vi "convertDeviceData.vi"   [LabVIEW 2011]
uses:
  GlobalVariables.vi
types:
  T1 = typedef "Device Cluster.ctl" = cluster{"Dnet":string, "Node":i32, "Type":string, "ID Number":u8, "SCCM":dbl, "FullScale":dbl, "Input Bytes":i32, "Output Bytes":i32, "Input Start Location":i32, "Output Start Location":i32, "Enabled":bool, "Bytes":u8[]}
  T2 = cluster{"[0]":u8, "[1]":u8, "[2]":u8, "[3]":u8, "[4]":u8, "[5]":u8, "[6]":u8, "[7]":u8}
  T3 = typedef "MFC Cluster.ctl" = cluster{"ID Number":u8, "Status":bool[], "Flow (SCCM)":dbl, "SetPoint (SCCM)":dbl, "Actuator Override":i8, "Actuator Drive Valve":i16, "Setpoint Output":dbl}
  T4 = typedef "PC Cluster.ctl" = cluster{"ID Number":u8, "Status":bool[], "Flow (SCCM)":dbl, "SetPoint (SCCM)":dbl, "Actuator Override":i8, "Actuator Drive Valve":i16, "Setpoint Output":dbl}
  T5 = typedef "RTPC Cluster.ctl" = cluster{"ID Number":u8, "Status":bool[], "Flow (SCCM)":dbl, "Pressure (SCCM)":dbl, "Valve":i16, "Active Instance":i8, "Output":dbl}
  T6 = typedef "GP275 Cluster.ctl" = cluster{"Pressure (Torr)":sgl}
  T7 = typedef "GP354 Cluster.ctl" = cluster{"Degas":bool, "Enable Filament 1":bool, "Enable Filament 2":bool, "Medium Emission":bool, "Ion Gauge":bool, "High Emission":bool, "Pressure":dbl}
  T8 = typedef "BAR Cluster.ctl" = cluster{"Pressure":dbl}
  T9 = typedef "EZ-ZONE Input Cluster.ctl" = cluster{"Device Status":u32, "Analog Input Value 1":sgl, "Analog Input Value 2":sgl, "Heat Power":sgl, "Cool Power":sgl, "Profile Start":u32, "Current Profile":u32, "Current Step":u32, "Active Set Point":sgl, "Step Time Remaining":u32, "Analog Input Error 1":u32, "Analog Input Error 2":u32, "Alarm State 1":u32, "Alarm State 2":u32, "Alarm State 3":u32, "Alarm State 4":u32, "Digital Input Status 5":u32, "Digital Input Status 6":u32, "Control Mode Active":u32, "Limit State":u32, "Profile Action Request":u32}
  T10 = typedef "EZ-ZONE Output Cluster.ctl" = cluster{"Loop Control Mode":u32, "Closed Loop Set Point":sgl, "Open Loop Set Point":sgl, "Alarm 1 - High Set Point":sgl, "Alarm 1 - Low Set Point":sgl, "Alarm 2 - High Set Point":sgl, "Alarm 2 - Low Set Point":sgl, "Alarm 3 - High Set Point":sgl, "Alarm 3 - Low Set Point":sgl, "Alarm 4 - High Set Point":sgl, "Alarm 4 - Low Set Point":sgl, "Profile Action Request":u32, "Profile Start":u32, "Heat Proportional Band":sgl, "Cool Proportional Band":sgl, "Time Integral":sgl, "Time Derivative":sgl, "Heat Hysteresis":sgl, "Cool Hysteresis":sgl, "Dead Band":sgl}
  T11 = typedef "TurboMotor Response Cluster.ctl" = cluster{"Enable":bool, "Index Level":bool, "Current Direction":bool, "General Fault":bool, "Profile in Progress":bool, "Load Complete":bool, "FE Fault":bool, "Rev Limit":bool, "Fwd Limit":bool, "Axis Number":u8, "Message Type":u16, "Data":u8[]}
  T12 = typedef "TurboMotor Command Cluster.ctl" = cluster{"Enable":bool, "Hard Stop":bool, "Smooth Stop":bool, "Direction":bool, "Incremental":bool, "Load Data/Start Profile":bool, "Axis Number":u8, "Message Type":u16, "Data":u8[]}
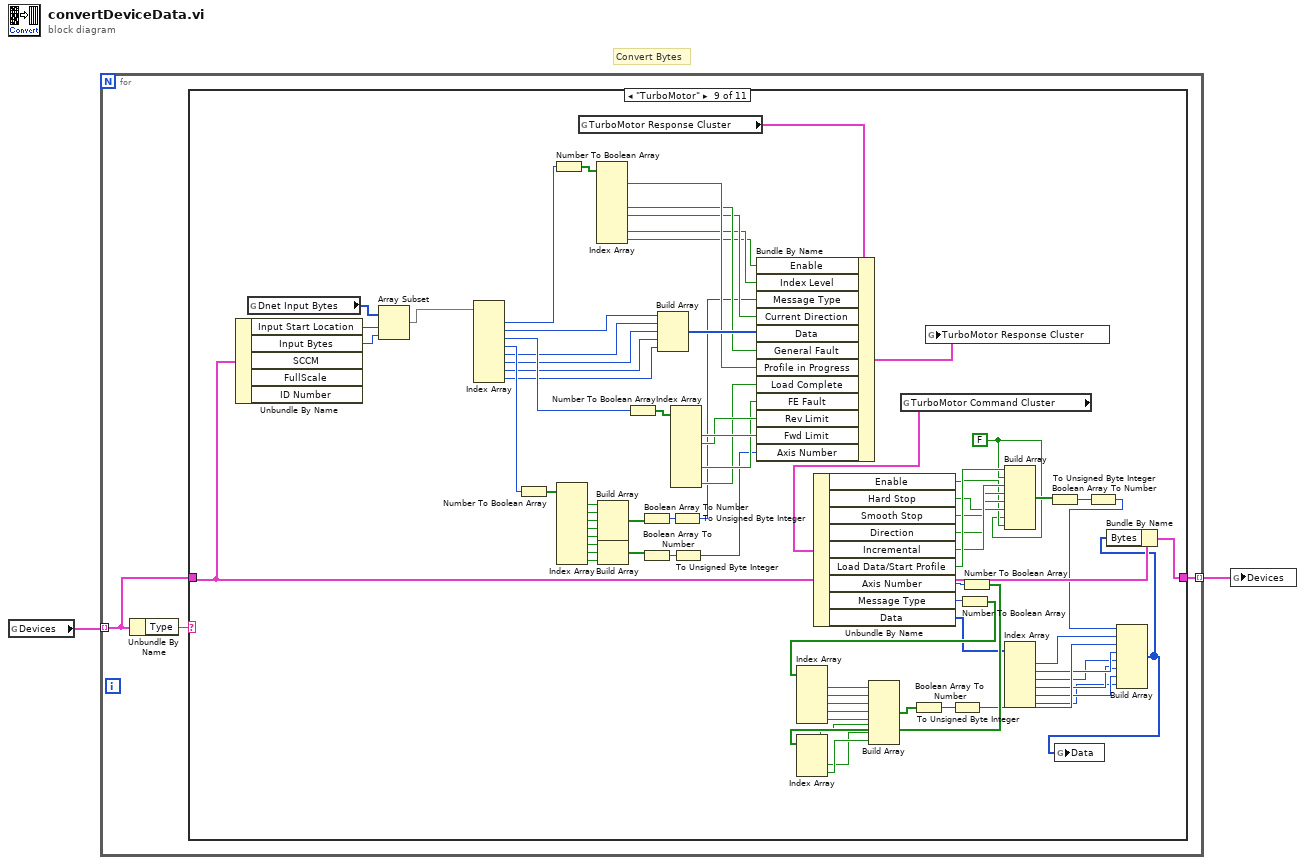
[diagram p0: block diagram]
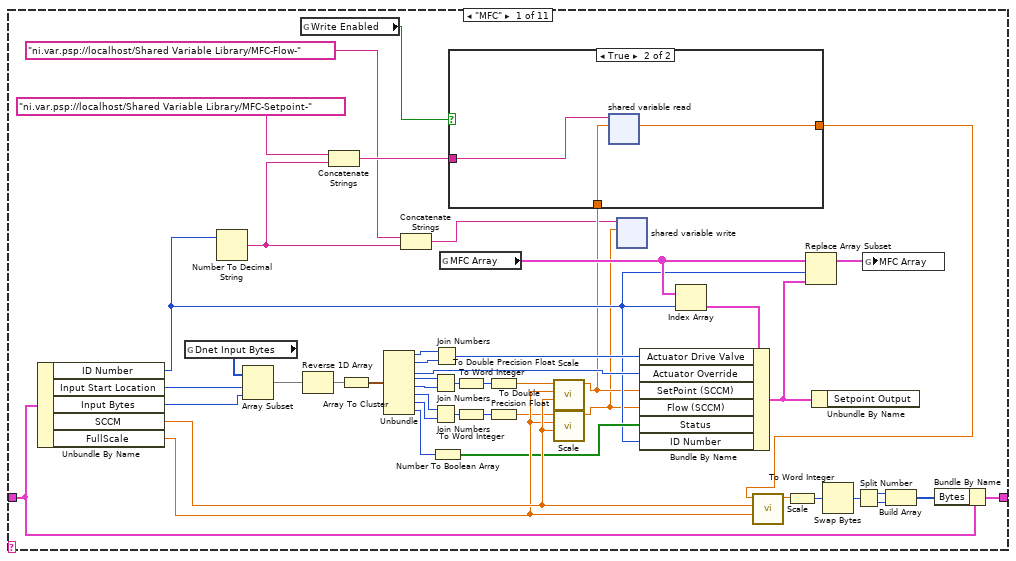
[diagram p2: hidden frame]
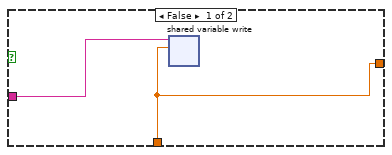
[diagram p3: hidden frame]
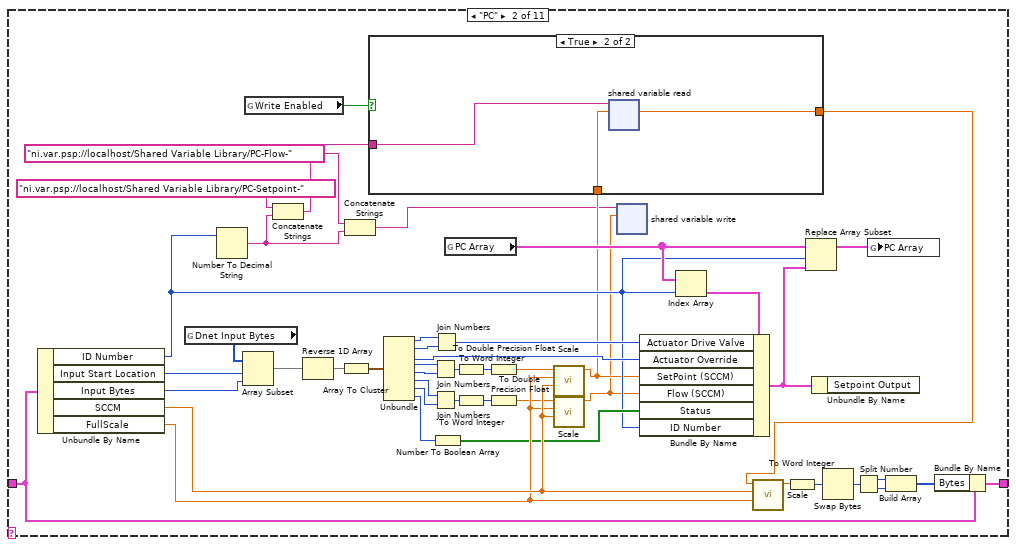
[diagram p4: hidden frame]
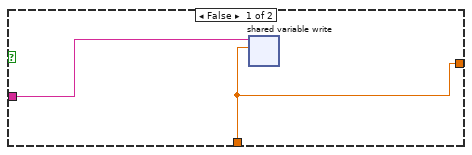
[diagram p5: hidden frame]
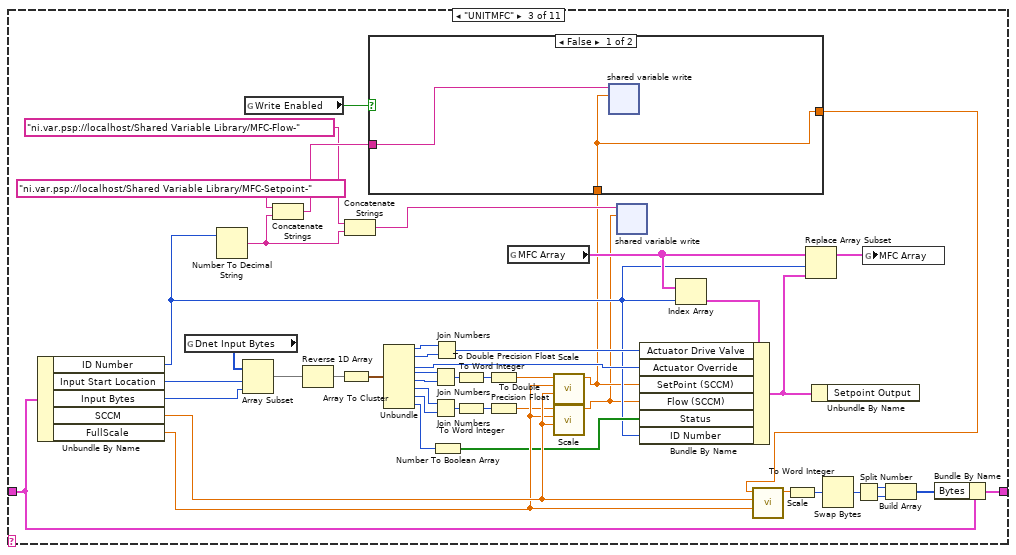
[diagram p6: hidden frame]
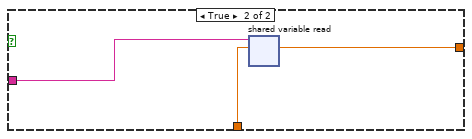
[diagram p7: hidden frame]
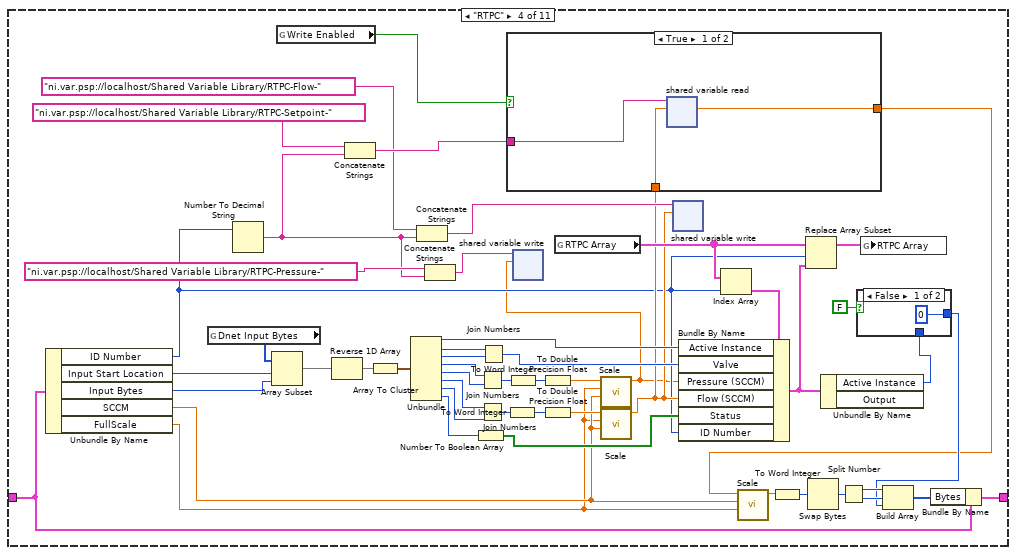
[diagram p8: hidden frame]
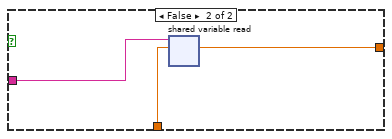
[diagram p9: hidden frame]
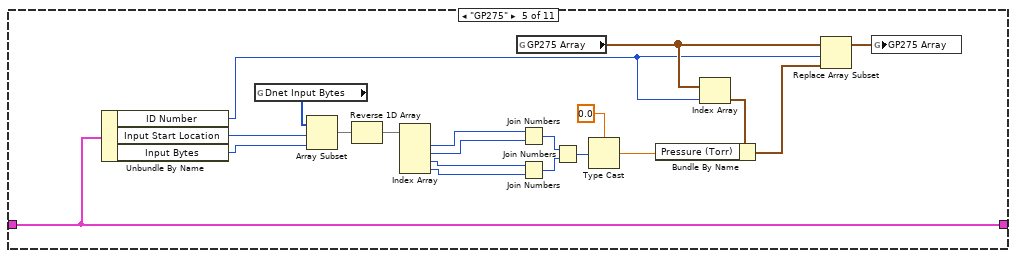
[diagram p11: hidden frame]
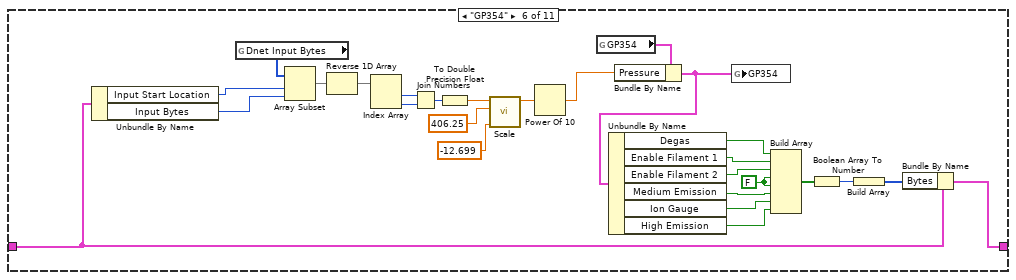
[diagram p12: hidden frame]
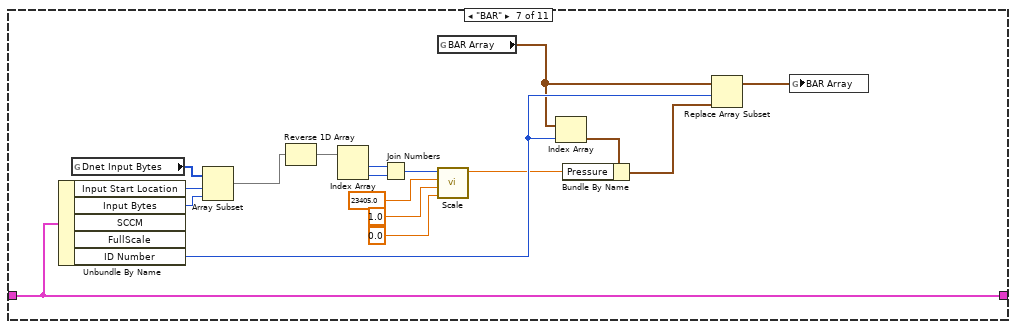
[diagram p13: hidden frame]
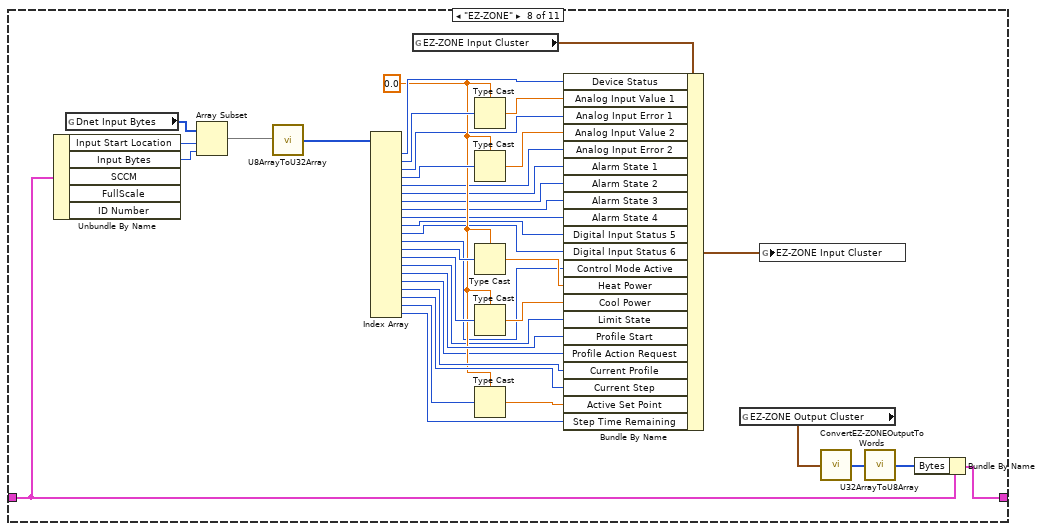
[diagram p14: hidden frame]
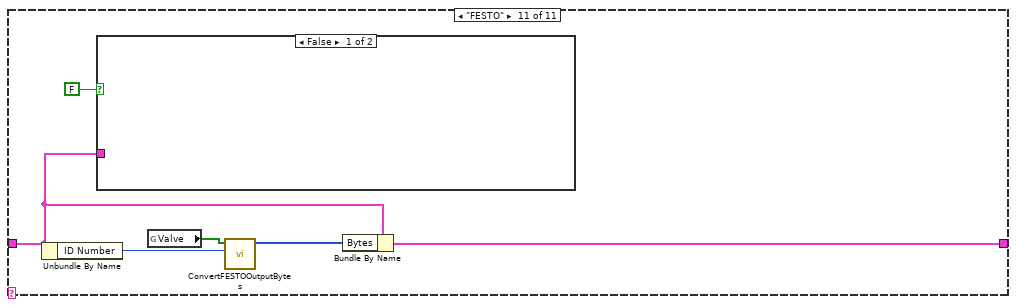
[diagram p16: hidden frame]
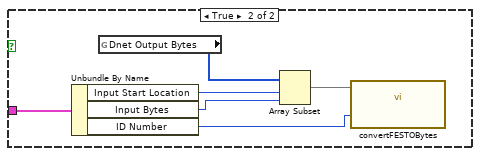
[diagram p17: hidden frame]
diagram:
  # "Convert Bytes"
  n1 = global read "GlobalVariables.vi" "Devices"() -> (w2:T1[])
  n2 = for {
    tunnel: w2 -> [w5] mode=indexing
    tunnel: [w3] -> w1 mode=indexing
    n3 = Unbundle By Name(w5) -> ("Type"=w4:string)
    n4 = case shown="\"TurboMotor\"" w4 {
      tunnel: w5 -> [w16 w67 w118 w174 w218 w262 w276 w283 w365 w399 w402]
      tunnel: [w17 w68 w119 w175 w218 w263 w276 w284 w364 w399 w401] -> w3
      frame "MFC" {
        n5 = Unbundle By Name(w16) -> ("ID Number"=w14:u8, "Input Start Location"=w51:i32, "Input Bytes"=w50:i32, "SCCM"=w49:dbl, "FullScale"=w48:dbl)
        n6 = global read "GlobalVariables.vi" "Dnet Input Bytes"() -> (w31:u8[])
        n7 = Number To Decimal String(number=w14) -> (decimal integer string=w8:string)  [unwired: 1 in]
        n8 = Array Subset(array=w31, index=w51, length=w50) -> (w32:u8[])
        n9 = global read "GlobalVariables.vi" "Write Enabled"() -> (w15:bool)
        n10 = Reverse 1D Array(array=w32) -> (reversed array=w19:u8[])
        n11 = Concatenate Strings("ni.var.psp://localhost/Shared Variable Library/MFC-Setpoint-", w8) -> (w12:string)
        n12 = Array To Cluster(array=w19) -> (cluster=w18:T2)
        n13 = Unbundle(w18) -> ("[0]"=w26:u8, "[1]"=w25:u8, "[2]"=w34:u8, "[3]"=w24:u8, "[4]"=w23:u8, "[5]"=w22:u8, "[6]"=w21:u8, "[7]"=w20:u8)
        n14 = Concatenate Strings("ni.var.psp://localhost/Shared Variable Library/MFC-Flow-", w8) -> (w7:string)
        n15 = Join Numbers(hi=w24, lo=w23) -> ((hi.lo)=w30:u16)
        n16 = Join Numbers(hi=w22, lo=w21) -> ((hi.lo)=w29:u16)
        n17 = Join Numbers(hi=w26, lo=w25) -> ((hi.lo)=w35:u16)
        n18 = Number To Boolean Array(number=w20) -> (Boolean array=w33:bool[])
        n19 = global read "GlobalVariables.vi" "MFC Array"() -> (w38:T3[])
        n20 = To Word Integer(number=w30) -> (16bit integer=w27:i16)
        n21 = To Word Integer(number=w29) -> (16bit integer=w28:i16)
        n22 = To Double Precision Float(number=w27) -> (double precision float=w40:dbl)
        n23 = To Double Precision Float(number=w28) -> (double precision float=w41:dbl)
        n24 = call "Scale.vi"("Factor"=w49, "FullScale"=w48, "Input"=w40) -> ("Output"=w11:dbl)  [unwired: 8 in]
        n25 = case shown="True" w15 {
          tunnel: w12 -> [w53 w56]
          tunnel: w11 -> [w52 w54]
          tunnel: [w52 w55] -> w10
          frame False {
            n26 = shared-variable-write(w53, w52) -> ()  [unwired: 1 in, 2 out]
          }
          frame True {
            n27 = shared-variable-read(w56, w54) -> (w55:dbl)  [unwired: 1 in, 3 out]
          }
        }
        n28 = call "Scale.vi"("Factor"=w49, "FullScale"=w48, "Input"=w41) -> ("Output"=w6:dbl)  [unwired: 8 in]
        n29 = shared-variable-write(w7, w6) -> ()  [unwired: 1 in, 2 out]
        n30 = Index Array(array=w38, index=w14) -> (element=w36:T3)
        n31 = Bundle By Name(cluster=w36, "Actuator Drive Valve"=w35, "Actuator Override"=w34, "SetPoint (SCCM)"=w11, "Flow (SCCM)"=w6, "Status"=w33, "ID Number"=w14) -> (w37:T3)
        n32 = call "Scale.vi"("Factor"=w48, "FullScale"=w49, "Input"=w10) -> ("Output"=w42:dbl)  [unwired: 8 in]
        n33 = To Word Integer(number=w42) -> (16bit integer=w43:i16)
        n34 = Replace Array Subset(array=w38, new element=w37, index=w14) -> (w39:T3[])
        n35 = Unbundle By Name(w37) -> ()  [unwired: 1 out]
        n36 = Swap Bytes(anything=w43) -> (byte swapped=w44:i16)
        n37 = Split Number(x=w44) -> (hi(x)=w46:u8, lo(x)=w45:u8)
        n38 = global write "GlobalVariables.vi" "MFC Array"(w39) -> ()
        n39 = Build Array(w46, w45) -> (w47:u8[])
        n40 = Bundle By Name(cluster=w16, "Bytes"=w47) -> (w17:T1)
      }
      frame "PC" {
        n41 = Unbundle By Name(w67) -> ("ID Number"=w65:u8, "Input Start Location"=w102:i32, "Input Bytes"=w101:i32, "SCCM"=w100:dbl, "FullScale"=w99:dbl)
        n42 = global read "GlobalVariables.vi" "Dnet Input Bytes"() -> (w82:u8[])
        n43 = Number To Decimal String(number=w65) -> (decimal integer string=w59:string)  [unwired: 1 in]
        n44 = Array Subset(array=w82, index=w102, length=w101) -> (w83:u8[])
        n45 = global read "GlobalVariables.vi" "Write Enabled"() -> (w66:bool)
        n46 = Concatenate Strings("ni.var.psp://localhost/Shared Variable Library/PC-Setpoint-", w59) -> (w63:string)
        n47 = Reverse 1D Array(array=w83) -> (reversed array=w70:u8[])
        n48 = Array To Cluster(array=w70) -> (cluster=w69:T2)
        n49 = Concatenate Strings("ni.var.psp://localhost/Shared Variable Library/PC-Flow-", w59) -> (w58:string)
        n50 = Unbundle(w69) -> ("[0]"=w77:u8, "[1]"=w76:u8, "[2]"=w85:u8, "[3]"=w75:u8, "[4]"=w74:u8, "[5]"=w73:u8, "[6]"=w72:u8, "[7]"=w71:u8)
        n51 = Join Numbers(hi=w75, lo=w74) -> ((hi.lo)=w81:u16)
        n52 = Join Numbers(hi=w73, lo=w72) -> ((hi.lo)=w80:u16)
        n53 = Join Numbers(hi=w77, lo=w76) -> ((hi.lo)=w86:u16)
        n54 = Number To Boolean Array(number=w71) -> (Boolean array=w84:bool[])
        n55 = global read "GlobalVariables.vi" "PC Array"() -> (w89:T4[])
        n56 = To Word Integer(number=w81) -> (16bit integer=w78:i16)
        n57 = To Word Integer(number=w80) -> (16bit integer=w79:i16)
        n58 = To Double Precision Float(number=w78) -> (double precision float=w91:dbl)
        n59 = To Double Precision Float(number=w79) -> (double precision float=w92:dbl)
        n60 = call "Scale.vi"("Factor"=w100, "FullScale"=w99, "Input"=w91) -> ("Output"=w62:dbl)  [unwired: 8 in]
        n61 = case shown="True" w66 {
          tunnel: w63 -> [w104 w107]
          tunnel: w62 -> [w103 w105]
          tunnel: [w103 w106] -> w61
          frame False {
            n62 = shared-variable-write(w104, w103) -> ()  [unwired: 1 in, 2 out]
          }
          frame True {
            n63 = shared-variable-read(w107, w105) -> (w106:dbl)  [unwired: 1 in, 3 out]
          }
        }
        n64 = call "Scale.vi"("Factor"=w100, "FullScale"=w99, "Input"=w92) -> ("Output"=w57:dbl)  [unwired: 8 in]
        n65 = shared-variable-write(w58, w57) -> ()  [unwired: 1 in, 2 out]
        n66 = Index Array(array=w89, index=w65) -> (element=w87:T4)
        n67 = Bundle By Name(cluster=w87, "Actuator Drive Valve"=w86, "Actuator Override"=w85, "SetPoint (SCCM)"=w62, "Flow (SCCM)"=w57, "Status"=w84, "ID Number"=w65) -> (w88:T4)
        n68 = call "Scale.vi"("Factor"=w99, "FullScale"=w100, "Input"=w61) -> ("Output"=w93:dbl)  [unwired: 8 in]
        n69 = To Word Integer(number=w93) -> (16bit integer=w94:i16)
        n70 = Replace Array Subset(array=w89, new element=w88, index=w65) -> (w90:T4[])
        n71 = Unbundle By Name(w88) -> ()  [unwired: 1 out]
        n72 = Swap Bytes(anything=w94) -> (byte swapped=w95:i16)
        n73 = Split Number(x=w95) -> (hi(x)=w97:u8, lo(x)=w96:u8)
        n74 = global write "GlobalVariables.vi" "PC Array"(w90) -> ()
        n75 = Build Array(w97, w96) -> (w98:u8[])
        n76 = Bundle By Name(cluster=w67, "Bytes"=w98) -> (w68:T1)
      }
      frame "UNITMFC" {
        n77 = Unbundle By Name(w118) -> ("ID Number"=w111:u8, "Input Start Location"=w153:i32, "Input Bytes"=w152:i32, "SCCM"=w151:dbl, "FullScale"=w150:dbl)
        n78 = global read "GlobalVariables.vi" "Dnet Input Bytes"() -> (w133:u8[])
        n79 = Number To Decimal String(number=w111) -> (decimal integer string=w113:string)  [unwired: 1 in]
        n80 = Array Subset(array=w133, index=w153, length=w152) -> (w134:u8[])
        n81 = global read "GlobalVariables.vi" "Write Enabled"() -> (w117:bool)
        n82 = Concatenate Strings("ni.var.psp://localhost/Shared Variable Library/MFC-Setpoint-", w113) -> (w115:string)
        n83 = Reverse 1D Array(array=w134) -> (reversed array=w121:u8[])
        n84 = Array To Cluster(array=w121) -> (cluster=w120:T2)
        n85 = Concatenate Strings("ni.var.psp://localhost/Shared Variable Library/MFC-Flow-", w113) -> (w112:string)
        n86 = Unbundle(w120) -> ("[0]"=w128:u8, "[1]"=w127:u8, "[2]"=w136:u8, "[3]"=w126:u8, "[4]"=w125:u8, "[5]"=w124:u8, "[6]"=w123:u8, "[7]"=w122:u8)
        n87 = Join Numbers(hi=w126, lo=w125) -> ((hi.lo)=w132:u16)
        n88 = Join Numbers(hi=w124, lo=w123) -> ((hi.lo)=w131:u16)
        n89 = Join Numbers(hi=w128, lo=w127) -> ((hi.lo)=w137:u16)
        n90 = Number To Boolean Array(number=w122) -> (Boolean array=w135:bool[])
        n91 = To Word Integer(number=w132) -> (16bit integer=w129:i16)
        n92 = To Word Integer(number=w131) -> (16bit integer=w130:i16)
        n93 = To Double Precision Float(number=w129) -> (double precision float=w142:dbl)
        n94 = To Double Precision Float(number=w130) -> (double precision float=w143:dbl)
        n95 = global read "GlobalVariables.vi" "MFC Array"() -> (w140:T3[])
        n96 = call "Scale.vi"("Factor"=w151, "FullScale"=w150, "Input"=w142) -> ("Output"=w110:dbl)  [unwired: 8 in]
        n97 = case shown="False" w117 {
          tunnel: w115 -> [w155 w158]
          tunnel: w110 -> [w154 w156]
          tunnel: [w154 w157] -> w108
          frame False {
            n98 = shared-variable-write(w155, w154) -> ()  [unwired: 1 in, 2 out]
          }
          frame True {
            n99 = shared-variable-read(w158, w156) -> (w157:dbl)  [unwired: 1 in, 3 out]
          }
        }
        n100 = call "Scale.vi"("Factor"=w151, "FullScale"=w150, "Input"=w143) -> ("Output"=w109:dbl)  [unwired: 8 in]
        n101 = shared-variable-write(w112, w109) -> ()  [unwired: 1 in, 2 out]
        n102 = Index Array(array=w140, index=w111) -> (element=w138:T3)
        n103 = Bundle By Name(cluster=w138, "Actuator Drive Valve"=w137, "Actuator Override"=w136, "SetPoint (SCCM)"=w110, "Flow (SCCM)"=w109, "Status"=w135, "ID Number"=w111) -> (w139:T3)
        n104 = call "Scale.vi"("Factor"=w150, "FullScale"=w151, "Input"=w108) -> ("Output"=w144:dbl)  [unwired: 8 in]
        n105 = To Word Integer(number=w144) -> (16bit integer=w145:i16)
        n106 = Replace Array Subset(array=w140, new element=w139, index=w111) -> (w141:T3[])
        n107 = Unbundle By Name(w139) -> ()  [unwired: 1 out]
        n108 = Swap Bytes(anything=w145) -> (byte swapped=w146:i16)
        n109 = Split Number(x=w146) -> (hi(x)=w148:u8, lo(x)=w147:u8)
        n110 = global write "GlobalVariables.vi" "MFC Array"(w141) -> ()
        n111 = Build Array(w148, w147) -> (w149:u8[])
        n112 = Bundle By Name(cluster=w118, "Bytes"=w149) -> (w119:T1)
      }
      frame "RTPC" {
        n113 = Unbundle By Name(w174) -> ("ID Number"=w163:u8, "Input Start Location"=w194:i32, "Input Bytes"=w195:i32, "SCCM"=w178:dbl, "FullScale"=w177:dbl)
        n114 = global read "GlobalVariables.vi" "Dnet Input Bytes"() -> (w197:u8[])
        n115 = Number To Decimal String(number=w163) -> (decimal integer string=w161:string)  [unwired: 1 in]
        n116 = Array Subset(array=w197, index=w194, length=w195) -> (w196:u8[])
        n117 = global read "GlobalVariables.vi" "Write Enabled"() -> (w166:bool)
        n118 = Reverse 1D Array(array=w196) -> (reversed array=w198:u8[])
        n119 = Concatenate Strings("ni.var.psp://localhost/Shared Variable Library/RTPC-Setpoint-", w161) -> (w170:string)
        n120 = Array To Cluster(array=w198) -> (cluster=w193:T2)
        n121 = Unbundle(w193) -> ("[0]"=w189:u8, "[1]"=w199:u8, "[2]"=w200:u8, "[3]"=w205:u8, "[4]"=w206:u8, "[5]"=w207:u8, "[6]"=w208:u8, "[7]"=w209:u8)
        n122 = Concatenate Strings("ni.var.psp://localhost/Shared Variable Library/RTPC-Flow-", w161) -> (w168:string)
        n123 = Concatenate Strings("ni.var.psp://localhost/Shared Variable Library/RTPC-Pressure-", w161) -> (w160:string)
        n124 = Number To Boolean Array(number=w209) -> (Boolean array=w188:bool[])
        n125 = Join Numbers(hi=w205, lo=w206) -> ((hi.lo)=w201:u16)
        n126 = Join Numbers(hi=w207, lo=w208) -> ((hi.lo)=w202:u16)
        n127 = Join Numbers(hi=w199, lo=w200) -> ((hi.lo)=w190:u16)
        n128 = To Word Integer(number=w202) -> (16bit integer=w203:i16)
        n129 = To Word Integer(number=w201) -> (16bit integer=w204:i16)
        n130 = To Double Precision Float(number=w204) -> (double precision float=w192:dbl)
        n131 = To Double Precision Float(number=w203) -> (double precision float=w191:dbl)
        n132 = global read "GlobalVariables.vi" "RTPC Array"() -> (w181:T5[])
        n133 = call "Scale.vi"("Factor"=w178, "FullScale"=w177, "Input"=w192) -> ("Output"=w159:dbl)  [unwired: 8 in]
        n134 = shared-variable-write(w160, w159) -> ()  [unwired: 1 in, 2 out]
        n135 = call "Scale.vi"("Factor"=w178, "FullScale"=w177, "Input"=w191) -> ("Output"=w165:dbl)  [unwired: 8 in]
        n136 = case shown="True" w166 {
          tunnel: w170 -> [w212 w215]
          tunnel: w165 -> [w210 w213]
          tunnel: [w211 w214] -> w164
          frame True {
            n137 = shared-variable-read(w212, w210) -> (w211:dbl)  [unwired: 1 in, 3 out]
          }
          frame False {
            n138 = shared-variable-read(w215, w213) -> (w214:dbl)  [unwired: 1 in, 3 out]
          }
        }
        n139 = shared-variable-write(w168, w165) -> ()  [unwired: 1 in, 2 out]
        n140 = Index Array(array=w181, index=w163) -> (element=w179:T5)
        n141 = Bundle By Name(cluster=w179, "Active Instance"=w189, "Valve"=w190, "Pressure (SCCM)"=w159, "Flow (SCCM)"=w165, "Status"=w188, "ID Number"=w163) -> (w176:T5)
        n142 = call "Scale.vi"("Factor"=w177, "FullScale"=w178, "Input"=w164) -> ("Output"=w187:dbl)  [unwired: 8 in]
        n143 = To Word Integer(number=w187) -> (16bit integer=w186:i16)
        n144 = Replace Array Subset(array=w181, new element=w176, index=w163) -> (w180:T5[])
        n145 = Swap Bytes(anything=w186) -> (byte swapped=w185:i16)
        n146 = Unbundle By Name(w176) -> ("Active Instance"=w173:i8)  [unwired: 1 out]
        n147 = Split Number(x=w185) -> (hi(x)=w183:u8, lo(x)=w184:u8)
        n148 = case shown="False" FALSE {
          tunnel: w173 -> [_ w217]
          tunnel: [0 w217] -> w172
          frame False {
          }
          frame True {
          }
        }
        n149 = global write "GlobalVariables.vi" "RTPC Array"(w180) -> ()
        n150 = Build Array(w183, w184, w172) -> (w182:i32[])
        n151 = Bundle By Name(cluster=w174, "Bytes"=w182) -> (w175:T1)
      }
      frame "GP275" {
        n152 = Unbundle By Name(w218) -> ("ID Number"=w219:u8, "Input Start Location"=w220:i32, "Input Bytes"=w221:i32)
        n153 = global read "GlobalVariables.vi" "Dnet Input Bytes"() -> (w233:u8[])
        n154 = Array Subset(array=w233, index=w220, length=w221) -> (w225:u8[])
        n155 = Reverse 1D Array(array=w225) -> (reversed array=w226:u8[])
        n156 = Index Array(array=w226) -> (element #1=w230:u8, element #2=w229:u8, element #3=w228:u8, element #4=w227:u8)  [unwired: 4 in]
        n157 = global read "GlobalVariables.vi" "GP275 Array"() -> (w223:T6[])
        n158 = Join Numbers(hi=w230, lo=w229) -> ((hi.lo)=w235:u16)
        n159 = Join Numbers(hi=w228, lo=w227) -> ((hi.lo)=w236:u16)
        n160 = Join Numbers(hi=w235, lo=w236) -> ((hi.lo)=w234:u32)
        n161 = Type Cast(type=sgl 0.0, x=w234) -> (*(type *) &x=w224:sgl)
        n162 = Index Array(array=w223, index=w219) -> (element=w232:T6)
        n163 = Bundle By Name(cluster=w232, "Pressure (Torr)"=w224) -> (w231:T6)
        n164 = Replace Array Subset(array=w223, new element=w231, index=w219) -> (w222:T6[])
        n165 = global write "GlobalVariables.vi" "GP275 Array"(w222) -> ()
      }
      frame "GP354" {
        w252 = FALSE
        n166 = Unbundle By Name(w262) -> ("Input Start Location"=w260:i32, "Input Bytes"=w261:i32)
        n167 = global read "GlobalVariables.vi" "Dnet Input Bytes"() -> (w264:u8[])
        n168 = Array Subset(array=w264, index=w260, length=w261) -> (w255:u8[])
        n169 = Reverse 1D Array(array=w255) -> (reversed array=w258:u8[])
        n170 = Index Array(array=w258) -> (element #1=w256:u8, element #2=w257:u8)  [unwired: 2 in]
        n171 = Join Numbers(hi=w256, lo=w257) -> ((hi.lo)=w259:u16)
        n172 = To Double Precision Float(number=w259) -> (double precision float=w243:dbl)
        n173 = call "Scale.vi"("Offset"=-12.699, "FullScale"=406.25, "Input"=w243) -> ("Output"=w240:dbl)  [unwired: 8 in]
        n174 = Power Of 10(x=w240) -> (10^x=w254:dbl)
        n175 = global read "GlobalVariables.vi" "GP354"() -> (w239:T7)
        n176 = Bundle By Name(cluster=w239, "Pressure"=w254) -> (w238:T7)
        n177 = Unbundle By Name(w238) -> ("Degas"=w250:bool, "Enable Filament 1"=w249:bool, "Enable Filament 2"=w248:bool, "Medium Emission"=w247:bool, "Ion Gauge"=w246:bool, "High Emission"=w245:bool)
        n178 = global write "GlobalVariables.vi" "GP354"(w238) -> ()
        n179 = Build Array(w250, w249, w248, w252, w252, w247, w246, w245) -> (w253:bool[])
        n180 = Boolean Array To Number(Boolean array=w253) -> (number=w251:u8)
        n181 = Build Array(w251) -> (w244:u8[])
        n182 = Bundle By Name(cluster=w262, "Bytes"=w244) -> (w263:T1)
      }
      frame "BAR" {
        n183 = Unbundle By Name(w276) -> ("Input Start Location"=w281:i32, "Input Bytes"=w280:i32, "ID Number"=w277:u8)  [unwired: 2 out]
        n184 = global read "GlobalVariables.vi" "Dnet Input Bytes"() -> (w282:u8[])
        n185 = Array Subset(array=w282, index=w281, length=w280) -> (w268:u8[])
        n186 = Reverse 1D Array(array=w268) -> (reversed array=w271:u8[])
        n187 = Index Array(array=w271) -> (element #1=w269:u8, element #2=w270:u8)  [unwired: 2 in]
        n188 = Join Numbers(hi=w269, lo=w270) -> ((hi.lo)=w275:u16)
        n189 = global read "GlobalVariables.vi" "BAR Array"() -> (w266:T8[])
        n190 = call "Scale.vi"("Offset"=0.0, "Factor"=1.0, "FullScale"=23405.0, "Input"=w275) -> ("Output"=w267:dbl)  [unwired: 7 in]
        n191 = Index Array(array=w266, index=w277) -> (element=w279:T8)
        n192 = Bundle By Name(cluster=w279, "Pressure"=w267) -> (w278:T8)
        n193 = Replace Array Subset(array=w266, new element=w278, index=w277) -> (w265:T8[])
        n194 = global write "GlobalVariables.vi" "BAR Array"(w265) -> ()
      }
      frame "EZ-ZONE" {
        w306 = sgl 0.0
        n195 = Unbundle By Name(w283) -> ("Input Start Location"=w292:i32, "Input Bytes"=w291:i32)  [unwired: 3 out]
        n196 = global read "GlobalVariables.vi" "Dnet Input Bytes"() -> (w290:u8[])
        n197 = Array Subset(array=w290, index=w292, length=w291) -> (w289:u8[])
        n198 = call "U8ArrayToU32Array.vi"("U8-bit Array"=w289) -> ("U32-bit Array"=w288:u32[])
        n199 = Index Array(array=w288) -> (element #1=w321:u32, element #2=w320:u32, element #3=w305:u32, element #4=w318:u32, element #5=w304:u32, element #6=w303:u32, element #7=w302:u32, element #8=w301:u32, element #9=w300:u32, element #10=w299:u32, element #11=w298:u32, element #12=w297:u32, element #13=w313:u32, element #14=w312:u32, element #15=w296:u32, element #16=w311:u32, element #17=w295:u32, element #18=w310:u32, element #19=w309:u32, element #20=w308:u32, element #21=w307:u32)  [unwired: 21 in]
        n200 = global read "GlobalVariables.vi" "EZ-ZONE Input Cluster"() -> (w294:T9)
        n201 = Type Cast(type=w306, x=w320) -> (*(type *) &x=w319:sgl)
        n202 = Type Cast(type=w306, x=w318) -> (*(type *) &x=w317:sgl)
        n203 = Type Cast(type=w306, x=w313) -> (*(type *) &x=w315:sgl)
        n204 = Type Cast(type=w306, x=w312) -> (*(type *) &x=w316:sgl)
        n205 = Type Cast(type=w306, x=w308) -> (*(type *) &x=w314:sgl)
        n206 = Bundle By Name(cluster=w294, "Device Status"=w321, "Analog Input Value 1"=w319, "Analog Input Error 1"=w305, "Analog Input Value 2"=w317, "Analog Input Error 2"=w304, "Alarm State 1"=w303, "Alarm State 2"=w302, "Alarm State 3"=w301, "Alarm State 4"=w300, "Digital Input Status 5"=w299, "Digital Input Status 6"=w298, "Control Mode Active"=w297, "Heat Power"=w315, "Cool Power"=w316, "Limit State"=w296, "Profile Start"=w311, "Profile Action Request"=w295, "Current Profile"=w310, "Current Step"=w309, "Active Set Point"=w314, "Step Time Remaining"=w307) -> (w293:T9)
        n207 = global read "GlobalVariables.vi" "EZ-ZONE Output Cluster"() -> (w285:T10)
        n208 = global write "GlobalVariables.vi" "EZ-ZONE Input Cluster"(w293) -> ()
        n209 = call "ConvertEZ-ZONEOutputToWords.vi"("EZ-ZONE Output Cluster"=w285) -> ("Word Array"=w286:u32[])
        n210 = call "U32ArrayToU8Array.vi"("U32-bit Array"=w286) -> ("U8-bit Array"=w287:u8[])
        n211 = Bundle By Name(cluster=w283, "Bytes"=w287) -> (w284:T1)
      }
      frame "TurboMotor" {
        w331 = FALSE
        n212 = Unbundle By Name(w365) -> ("Input Start Location"=w396:i32, "Input Bytes"=w397:i32)  [unwired: 3 out]
        n213 = global read "GlobalVariables.vi" "Dnet Input Bytes"() -> (w398:u8[])
        n214 = Array Subset(array=w398, index=w396, length=w397) -> (w392:u8[])
        n215 = Index Array(array=w392) -> (element #1=w330:u8, element #2=w329:u8, element #3=w328:u8, element #4=w327:u8, element #5=w326:u8, element #6=w325:u8, element #7=w324:u8, element #8=w323:u8)  [unwired: 8 in]
        n216 = Number To Boolean Array(number=w327) -> (Boolean array=w380:bool[])
        n217 = Number To Boolean Array(number=w330) -> (Boolean array=w391:bool[])
        n218 = Index Array(array=w380) -> (element #1=w379:bool, element #2=w378:bool, element #3=w377:bool, element #4=w376:bool, element #5=w375:bool, element #6=w372:bool, element #7=w373:bool, element #8=w374:bool)  [unwired: 8 in]
        n219 = global read "GlobalVariables.vi" "TurboMotor Response Cluster"() -> (w395:T11)
        n220 = Index Array(array=w391) -> (element #1=w390:bool, element #4=w389:bool, element #5=w388:bool, element #7=w387:bool, element #8=w386:bool)  [unwired: 8 in, 3 out]
        n221 = Build Array(w379, w378, w377, w376, w375) -> (w371:bool[])
        n222 = Build Array(w372, w373, w374) -> (w370:bool[])
        n223 = Number To Boolean Array(number=w328) -> (Boolean array=w385:bool[])
        n224 = Boolean Array To Number(Boolean array=w371) -> (number=w368:u32)
        n225 = Boolean Array To Number(Boolean array=w370) -> (number=w369:u32)
        n226 = Build Array(w329, w326, w325, w324, w323) -> (w393:u8[])
        n227 = Index Array(array=w385) -> (element #2=w384:bool, element #3=w383:bool, element #6=w382:bool, element #8=w381:bool)  [unwired: 8 in, 4 out]
        n228 = To Unsigned Byte Integer(number=w368) -> (unsigned 8bit integer=w367:u8)
        n229 = To Unsigned Byte Integer(number=w369) -> (unsigned 8bit integer=w366:u8)
        n230 = Bundle By Name(cluster=w395, "Enable"=w386, "Index Level"=w387, "Message Type"=w367, "Current Direction"=w388, "Data"=w393, "General Fault"=w389, "Profile in Progress"=w390, "Load Complete"=w381, "FE Fault"=w382, "Rev Limit"=w383, "Fwd Limit"=w384, "Axis Number"=w366) -> (w394:T11)
        n231 = global read "GlobalVariables.vi" "TurboMotor Command Cluster"() -> (w363:T12)
        n232 = Unbundle By Name(w363) -> ("Enable"=w357:bool, "Hard Stop"=w358:bool, "Smooth Stop"=w359:bool, "Direction"=w360:bool, "Incremental"=w361:bool, "Load Data/Start Profile"=w362:bool, "Axis Number"=w353:u8, "Message Type"=w354:u16, "Data"=w340:u8[])
        n233 = global write "GlobalVariables.vi" "TurboMotor Response Cluster"(w394) -> ()
        n234 = Number To Boolean Array(number=w354) -> (Boolean array=w352:bool[])
        n235 = Index Array(array=w352) -> (element #1=w343:bool, element #2=w344:bool, element #3=w345:bool, element #4=w346:bool, element #5=w347:bool)  [unwired: 5 in]
        n236 = Number To Boolean Array(number=w353) -> (Boolean array=w351:bool[])
        n237 = Index Array(array=w351) -> (element #1=w348:bool, element #2=w349:bool, element #3=w350:bool)  [unwired: 3 in]
        n238 = Build Array(w343, w344, w345, w346, w347, w348, w349, w350) -> (w341:bool[])
        n239 = Boolean Array To Number(Boolean array=w341) -> (number=w342:u32)
        n240 = To Unsigned Byte Integer(number=w342) -> (unsigned 8bit integer=w337:u8)
        n241 = Build Array(w362, w331, w361, w360, w359, w358, w331, w357) -> (w356:bool[])
        n242 = Index Array(array=w340) -> (element #1=w338:u8, element #2=w336:u8, element #3=w335:u8, element #4=w334:u8, element #5=w333:u8, element #6=w332:u8)  [unwired: 6 in]
        n243 = Boolean Array To Number(Boolean array=w356) -> (number=w355:u32)
        n244 = To Unsigned Byte Integer(number=w355) -> (unsigned 8bit integer=w339:u8)
        n245 = Build Array(w339, w338, w337, w336, w335, w334, w333, w332) -> (w322:u8[])
        n246 = global write "GlobalVariables.vi" "Data"(w322) -> ()
        n247 = Bundle By Name(cluster=w365, "Bytes"=w322) -> (w364:T1)
      }
      frame "Undefined", Default {
      }
      frame "FESTO" {
        n248 = Unbundle By Name(w402) -> ("ID Number"=w404:u8)
        n249 = case shown="False" FALSE {
          tunnel: w402 -> [_ w408]
          frame False {
          }
          frame True {
            n250 = Unbundle By Name(w408) -> ("Input Start Location"=w410:i32, "Input Bytes"=w409:i32, "ID Number"=w406:u8)
            n251 = global read "GlobalVariables.vi" "Dnet Output Bytes"() -> (w411:u8[])
            n252 = Array Subset(array=w411, index=w410, length=w409) -> (w407:u8[])
            n253 = call "convertFESTOBytes.vi"("ID Number"=w406, "Bytes"=w407) -> ()  [unwired: 10 in]
          }
        }
        n254 = global read "GlobalVariables.vi" "Valve"() -> (w403:bool[])
        n255 = call "ConvertFESTOOutputBytes.vi"("Festo Block"=w404, "Valves"=w403) -> ("Bytes"=w400:u8[])  [unwired: 9 in]
        n256 = Bundle By Name(cluster=w402, "Bytes"=w400) -> (w401:T1)
      }
    }
  }
  n257 = global write "GlobalVariables.vi" "Devices"(w1) -> ()
